vi "CTRE_PigeonIMU_Open_CAN.vi"(8 "error in":errorcluster, 10 "Device Number":u8) -> (0 "error out":errorcluster, 3 "PigeonIMUDevRef":T1={"DeviceStatus"={"status"=FALSE, "code"=0, "source"=""}, "Device Number"=0, "Type"=352321536, "Device ID"=0, "Handle"=0, "UsageFrame"=0, "Library Path"=path ""} {"Type" items=["CAN"=352321536, "TalonSRX"=33554432]})   [LabVIEW 2017]
doc: "Opens a Pigeon IMU Device Reference using a CAN ID."
uses:
  CTRE_PigeonIMU_DeviceRef.ctl
  CTRE_PigeonIMU_ConnectionType.ctl
  <vilib>/Rock Robotics/SystemInterfaces/NetworkCommunication/NetComm_UsageReport_ResourceType.ctl
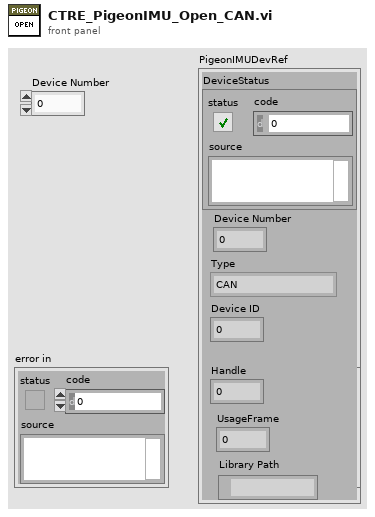
[diagram p1: front panel]
types:
  T1 = typedef "CTRE_PigeonIMU_DeviceRef.ctl" = cluster{"DeviceStatus":errorcluster, "Device Number":u8, "Type":T2, "Device ID":u32, "Handle":u64, "UsageFrame":u32, "Library Path":path}
  T2 = typedef "CTRE_PigeonIMU_ConnectionType.ctl" = u32
  T3 = typedef "NetComm_UsageReport_ResourceType.ctl" = enum8{"Controller", "Module", "Language", "CANPlugin", "Accelerometer", "ADXL345", "AnalogChannel", "AnalogTrigger", "AnalogTriggerOutput", "CANJaguar", "Compressor", "Counter", "Dashboard", "DigitalInput", "DigitalOutput", "DriverStationCIO", "DriverStationEIO", "DriverStationLCD", "Encoder", "GearTooth", "Gyro", "I2C", "Framework", "Jaguar", "Joystick", "Kinect", "KinectStick", "PIDController", "Preferences", "PWM", "Relay", "RobotDrive", "SerialPort", "Servo", "Solenoid", "SPI", "Task", "Ultrasonic", "Victor", "Button", "Command", "AxisCamera", "PCVideoServer", "SmartDashboard", "Talon", "HiTechnicColorSensor", "HiTechnicAccel", "HiTechnicCompass", "SRF08", "AnalogOutput", "Victor SP", "Talon SRX", "CAN Talon SRX", "ADXL362 Accel", "ADXRS450 Gyro", "Rev SPARK", "Mindsensors SD540", "Digital Filter", "ADIS16448", "PDP", "PCM", "PigeonIMU", "Nidec Brushless", "CTRE CANifier", "CTRE Future 0", "CTRE Future 1", "CTRE Future 2", "CTRE Future 3", "CTRE Future 4", "CTRE Future 5", "CTRE Future 6"}
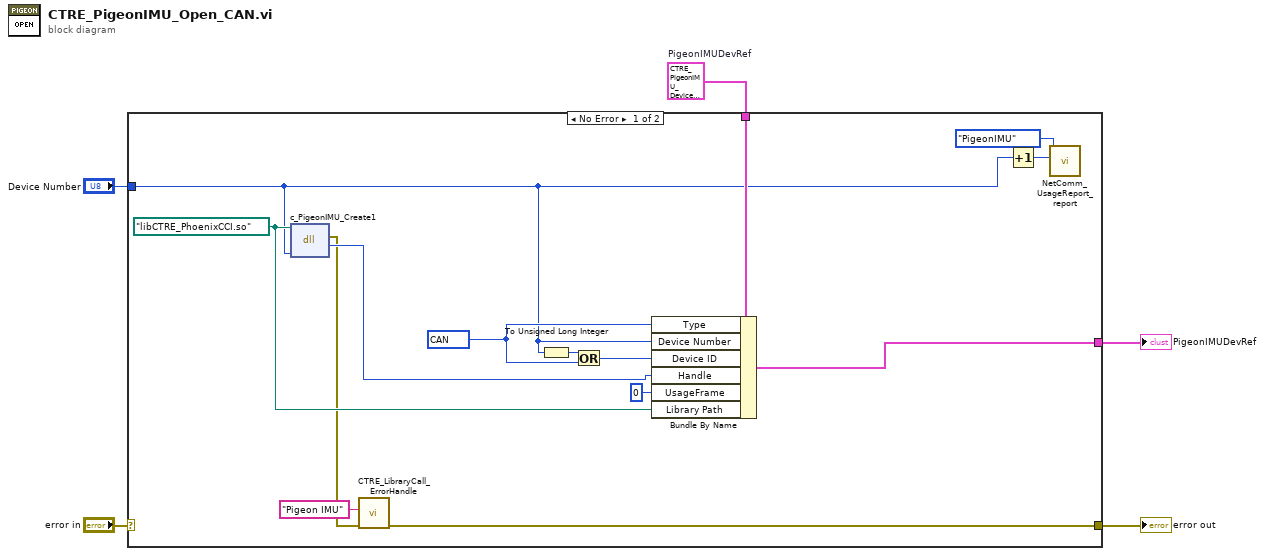
[diagram p0: block diagram]
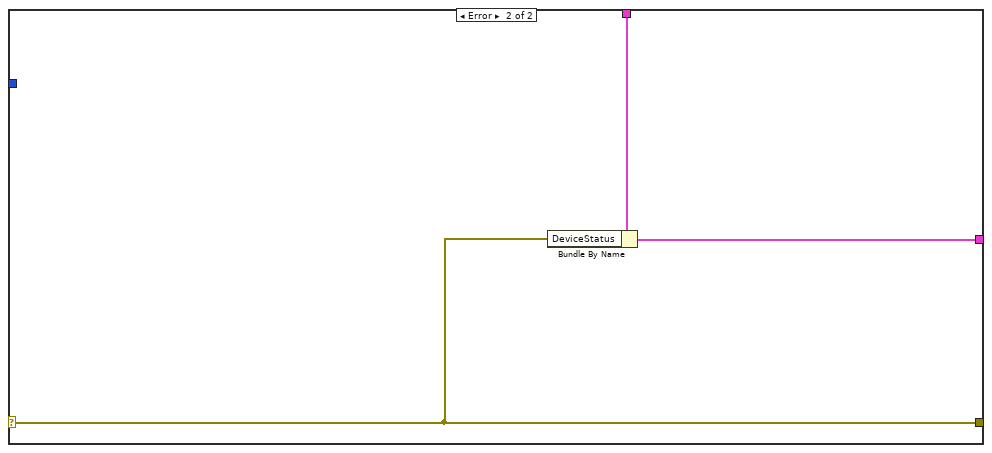
[diagram p2: hidden frame]
diagram:
  w3 = T1 {"DeviceStatus"={"status"=FALSE, "code"=0, "source"=""}, "Device Number"=0, "Type"=352321536, "Device ID"=0, "Handle"=0, "UsageFrame"=0, "Library Path"=path ""}  # PigeonIMUDevRef
  n1 = case shown="No Error" "error in" {
    selector: "error in" -> [_ w21]
    tunnel: [w12 w21] -> w4
    tunnel: w3 -> [w19 w22]
    tunnel: [w9 w20] -> w2
    tunnel: "Device Number" -> [w6 _]
    frame No Error {
      w15 = path "libCTRE_PhoenixCCI.so" ("path in")
      w16 = T2 352321536 items=["CAN"=352321536, "TalonSRX"=33554432] ("Connection Type")
      n2 = dll-call lib="?" fn="c_PigeonIMU_Create1"(path in=w15, "deviceNumber"=w6) -> (error out=w11:errorcluster, "return type"=w14:u64)  [unwired: 3 in, 1 out]
      n3 = call "CTRE_LibraryCall_ErrorHandle.vi"("error in"=w11, "DeviceType"="Pigeon IMU") -> ("error out"=w12:errorcluster)  [unwired: 9 in]
      n4 = To Unsigned Long Integer(number=w6) -> (unsigned 32bit integer=w18:u32)
      n5 = Or(x=w18, y=w16) -> (x .or. y?=w17:T2)
      n6 = Bundle By Name(cluster=w19, "Type"=w16, "Device Number"=w6, "Device ID"=w17, "Handle"=w14, "UsageFrame"=u32 0, "Library Path"=w15) -> (w9:T1)
      n7 = Increment(x=w6) -> (x+1=w8:u8)
      n8 = call <vilib>:"NetComm_UsageReport_report.vi"("Instance Number"=w8, "Resource Type"=NetComm_UsageReport_ResourceType."PigeonIMU") -> ()  [unwired: 10 in]
    }
    frame Error {
      n9 = Bundle By Name(cluster=w22, "DeviceStatus"=w21) -> (w20:T1)
    }
  }
  "error out" <- w4
  "PigeonIMUDevRef" <- w2
